vi "Counter - Read Pulse Width and Frequency (Continuous).vi"() -> ()   [LabVIEW 2022 SP3]
doc: "This example demonstrates how to continuously perform period, frequency, pulse width, or two edge separation measurement types.\n\nThis example uses implicit timing, which means that a sample is acquired for every period of your input signal.\n\nFor instructions on how to connect your signals to the DAQ device, refer to your device documentation."
uses:
  <vilib>/Utility/error.llb/DialogType.ctl
  <vilib>/DAQmx/read.llb/DAQmx Read (Counter 1D DBL 1Chan NSamp).vi
  <vilib>/DAQmx/create/channels.llb/DAQmx Create Channel (CI-Period).vi
  <vilib>/DAQmx/create/channels.llb/DAQmx Create Channel (CI-Frequency).vi
  <vilib>/DAQmx/create/channels.llb/DAQmx Create Channel (CI-Pulse Width).vi
  <vilib>/DAQmx/create/channels.llb/DAQmx Create Channel (CI-Two Edge Separation).vi
  <vilib>/DAQmx/configure/timing.llb/DAQmx Timing (Implicit).vi
  <vilib>/DAQmx/miscellaneous.llb/DAQmx Fill In Error Info.vi
  <resource>/objmgr/daqmx.rc
panel:
  out "Data":dbl[](array[numeric])
  in  "Counter Input Type":T1(tab)
  in  "Period Input Terminal":tag="/Dev1/PFI9"
  in  "Max Period":dbl=0.1 format="%0.6f"
  in  "Min Period":dbl=1e-06 format="%0.6f"
  in  "Min Frequency":dbl=2.0 format="%0.6f"
  in  "Max Frequency":dbl=100.0 format="%0.6f"
  in  "Frequency Input Terminal":tag="/Dev1/PFI9"
  in  "Pulse Width Input Terminal":tag="/Dev1/PFI9"
  in  "Min Pulse Width":dbl=1e-06 format="%0.6f"
  in  "Max Pulse Width":dbl=0.1 format="%0.6f"
  in  "Second Input Terminal":tag="/Dev1/PFI9"
  in  "Frst Input Terminal":tag="/Dev1/PFI10"
  in  "Min Separation Time":dbl=1e-06 format="%0.6f"
  in  "Max Separation Time":dbl=0.1 format="%0.6f"
  in  "Stop":bool
  in  "Samples per Loop":i32=1000
  in  "Counter":tag="Dev1/ctr0"
  # "Channel Settings"
  # "Acquired Data"
  # "Timing Settings"
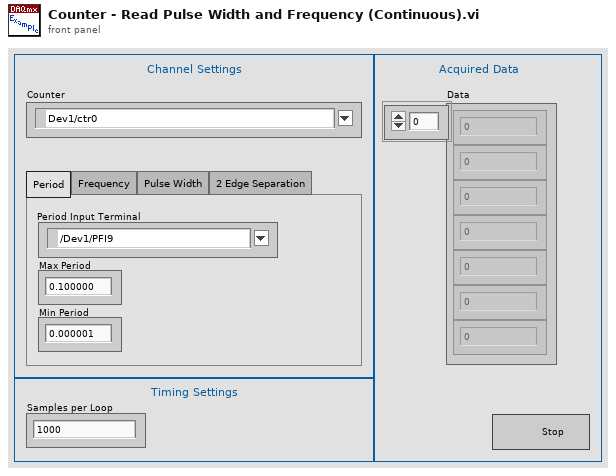
[diagram p1: front panel]
types:
  T1 = enum32{"Period", "Frequency", "Pulse Width", "2 Edge Separation"}
  T2 = typedef "DialogType.ctl" = u16
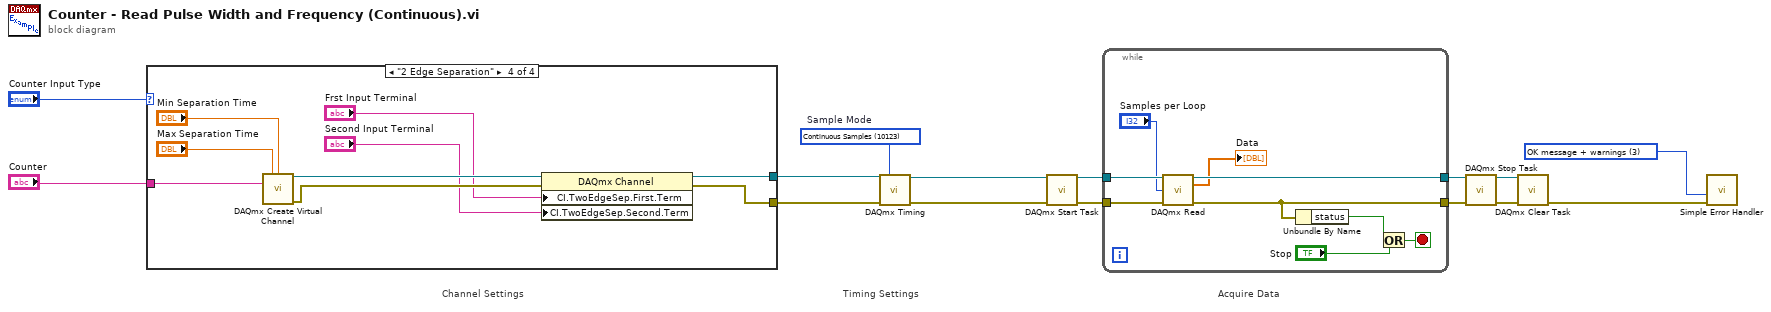
[diagram p0: block diagram]
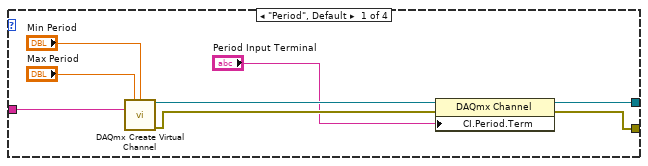
[diagram p2: hidden frame]
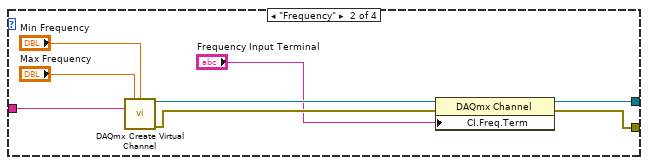
[diagram p3: hidden frame]
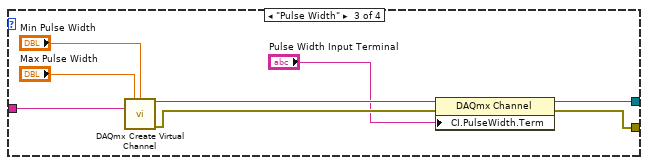
[diagram p4: hidden frame]
diagram:
  w1 = T2 3 items=["no dialog", "OK message", "continue or stop message", "OK message + warnings", "continue/stop + warnings"] ("type of dialog (OK msg:1)")
  w15 = 10123 items=["Finite Samples"=10178, "Continuous Samples"=10123, "Hardware Timed Single Point"=12522]  # Sample Mode
  # "Acquire Data"
  # "Timing Settings"
  # "Channel Settings"
  n1 = case shown="\"2 Edge Separation\"" "Counter Input Type" {
    tunnel: [w21 w29 w37 w46] -> w14
    tunnel: [w22 w30 w38 w47] -> w13
    tunnel: "Counter" -> [w23 w31 w39 w48]
    frame "Period", Default {
      n2 = call-poly <vilib>:"DAQmx Create Virtual Channel.vi"("maximum value"="Max Period", "minimum value"="Min Period", "counter"=w23) -> ("task out"=w20:refnum<k21>, "error out"=w19:errorcluster)  [unwired: 11 in]
      n3 = property class="DAQmx Channel"(reference=w20, error in=w19, "CI.Period.Term"="Period Input Terminal") -> (reference out=w22:refnum<k21>, error out=w21:errorcluster)
    }
    frame "Frequency" {
      n4 = call-poly <vilib>:"DAQmx Create Virtual Channel.vi"("maximum value"="Max Frequency", "minimum value"="Min Frequency", "counter"=w31) -> ("task out"=w28:refnum<k21>, "error out"=w27:errorcluster)  [unwired: 11 in]
      n5 = property class="DAQmx Channel"(reference=w28, error in=w27, "CI.Freq.Term"="Frequency Input Terminal") -> (reference out=w30:refnum<k21>, error out=w29:errorcluster)
    }
    frame "Pulse Width" {
      n6 = call-poly <vilib>:"DAQmx Create Virtual Channel.vi"("maximum value"="Max Pulse Width", "minimum value"="Min Pulse Width", "counter"=w39) -> ("task out"=w36:refnum<k21>, "error out"=w35:errorcluster)  [unwired: 11 in]
      n7 = property class="DAQmx Channel"(reference=w36, error in=w35, "CI.PulseWidth.Term"="Pulse Width Input Terminal") -> (reference out=w38:refnum<k21>, error out=w37:errorcluster)
    }
    frame "2 Edge Separation" {
      n8 = call-poly <vilib>:"DAQmx Create Virtual Channel.vi"("maximum value"="Max Separation Time", "minimum value"="Min Separation Time", "counter"=w48) -> ("task out"=w45:refnum<k21>, "error out"=w44:errorcluster)  [unwired: 11 in]
      n9 = property class="DAQmx Channel"(reference=w45, error in=w44, "CI.TwoEdgeSep.First.Term"="Frst Input Terminal", "CI.TwoEdgeSep.Second.Term"="Second Input Terminal") -> (reference out=w47:refnum<k21>, error out=w46:errorcluster)
    }
  }
  n10 = call-poly <vilib>:"DAQmx Timing.vi"("task/channels in"=w13, "sample mode"=w15, "error in"=w14) -> ("task out"=w7:refnum<k21>, "error out"=w6:errorcluster)  [unwired: 11 in]
  n11 = call <vilib>:"DAQmx Start Task.vi"("task/channels in"=w7, "error in"=w6) -> ("task out"=w12:refnum<k21>, "error out"=w11:errorcluster)  [unwired: 12 in]
  n12 = while {
    tunnel: w12 -> [w57]
    tunnel: w11 -> [w56]
    tunnel: [w53] -> w2
    tunnel: [w54] -> w3
    stop <- w55 stop-if-true
    n13 = call-poly <vilib>:"DAQmx Read.vi"("task/channels in"=w57, "number of samples per channel"="Samples per Loop", "error in"=w56) -> ("task out"=w54:refnum<k21>, "data"=→"Data":dbl[], "error out"=w53:errorcluster)  [unwired: 10 in]
    n14 = Unbundle By Name(w53) -> ("status"=w52:bool)
    n15 = Or(x=w52, y="Stop") -> (x .or. y?=w55:bool)
  }
  n16 = call <vilib>:"DAQmx Stop Task.vi"("task/channels in"=w3, "error in"=w2) -> ("task out"=w5:refnum<k21>, "error out"=w4:errorcluster)  [unwired: 12 in]
  n17 = call <vilib>:"DAQmx Clear Task.vi"("task in"=w5, "error in"=w4) -> ("error out"=w10:errorcluster)  [unwired: 13 in]
  n18 = call <vilib>:"Simple Error Handler.vi"("type of dialog (OK msg:1)"=w1, "error in (no error)"=w10) -> ()  [unwired: 3 in, 5 out]
